vi "e-block.vi"(0 "Strings in":string[](array[string]), 1 "Dubs in":dbl[](array[numeric])) -> ()   [LabVIEW 2018]
uses:
  <vilib>/DAQmx/write.llb/DAQmx Write (Analog DBL 1Chan 1Samp).vi
  <vilib>/DAQmx/create/channels.llb/DAQmx Create Channel (AO-Voltage-Basic).vi
  <vilib>/DAQmx/miscellaneous.llb/DAQmx Fill In Error Info.vi
panel:
  in  "subvi":bool=TRUE
  out "error out":errorcluster
  in  "AO2 name":string="6723"
  in  "e-block ao line":string="/ao0"
  in  "ON voltage":dbl=1.5 format="%#_13g"
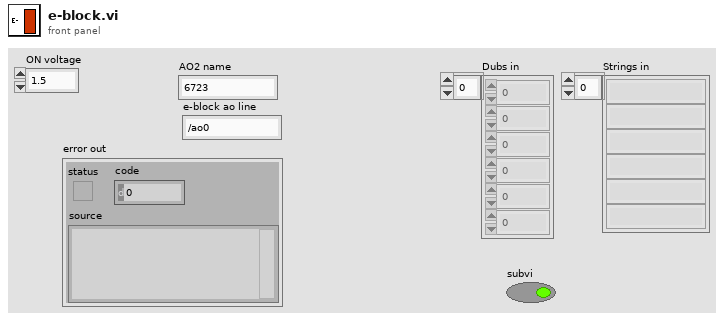
[diagram p1: front panel]
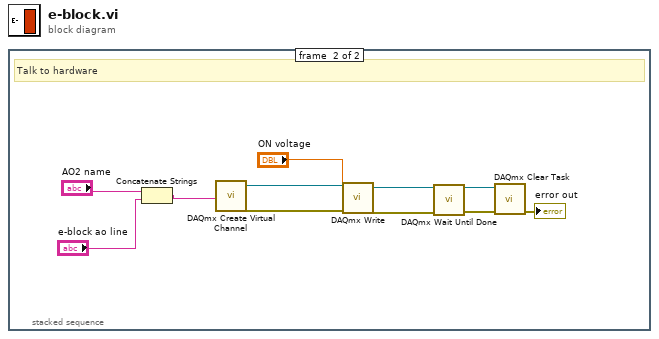
[diagram p0: block diagram]
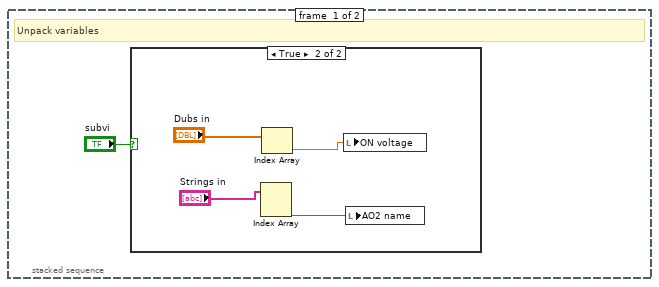
[diagram p2: hidden frame]
diagram:
  n1 = stacked-sequence {
    frame #0 {
      # "Unpack variables"
      n2 = case shown="True" "subvi" {
        frame False {
        }
        frame True {
          n3 = Index Array(array="Strings in") -> (element #2=w2:string)  [unwired: 2 in, 1 out]
          n4 = Index Array(array="Dubs in") -> (element=w3:dbl)  [unwired: 1 in]
          n5 = local write "ON voltage"(w3) -> ()
          n6 = local write "AO2 name"(w2) -> ()
        }
      }
    }
    frame #1 {
      # "Talk to hardware"
      n7 = Concatenate Strings("AO2 name", "e-block ao line") -> (w10:string)
      n8 = call-poly <vilib>:"DAQmx Create Virtual Channel.vi"("physical channels"=w10) -> ("task out"=w16:refnum<k21>, "error out"=w15:errorcluster)  [unwired: 13 in]
      n9 = call-poly <vilib>:"DAQmx Write.vi"("task/channels in"=w16, "data"="ON voltage", "error in"=w15) -> ("task out"=w12:refnum<k21>, "error out"=w11:errorcluster)  [unwired: 10 in, 1 out]
      n10 = call <vilib>:"DAQmx Wait Until Done.vi"("task/channels in"=w12, "error in"=w11) -> ("task out"=w14:refnum<k21>, "error out"=w13:errorcluster)  [unwired: 12 in]
      n11 = call <vilib>:"DAQmx Clear Task.vi"("task in"=w14, "error in"=w13) -> ("error out"=→"error out":errorcluster)  [unwired: 13 in]
    }
  }
